vi "gen_logstring.vi"(11 "Movelist":T1[](array[typedef])) -> (3 "LogString":string)   [LabVIEW 2015]
uses:
  chess_moveinfo_cluster.ctl
  chess_piecetype_enum.ctl
  chess_teamcolor_enum.ctl
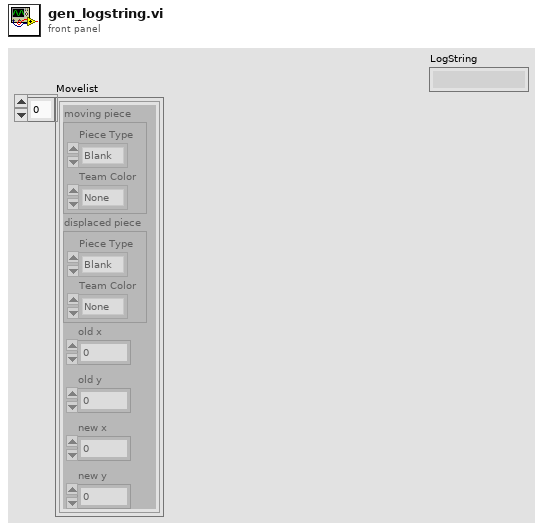
[diagram p1: front panel]
types:
  T1 = typedef "chess_moveinfo_cluster.ctl" = cluster{"moving piece":cluster{"Piece Type":T2, "Team Color":T3}, "displaced piece":cluster{"Piece Type":T2, "Team Color":T3}, "old x":i32, "old y":i32, "new x":i32, "new y":i32}
  T2 = typedef "chess_piecetype_enum.ctl" = enum16{"Blank", "Pawn", "Rook", "Knight", "Bishop", "Queen", "King"}
  T3 = typedef "chess_teamcolor_enum.ctl" = enum16{"None", "Red", "Blue"}
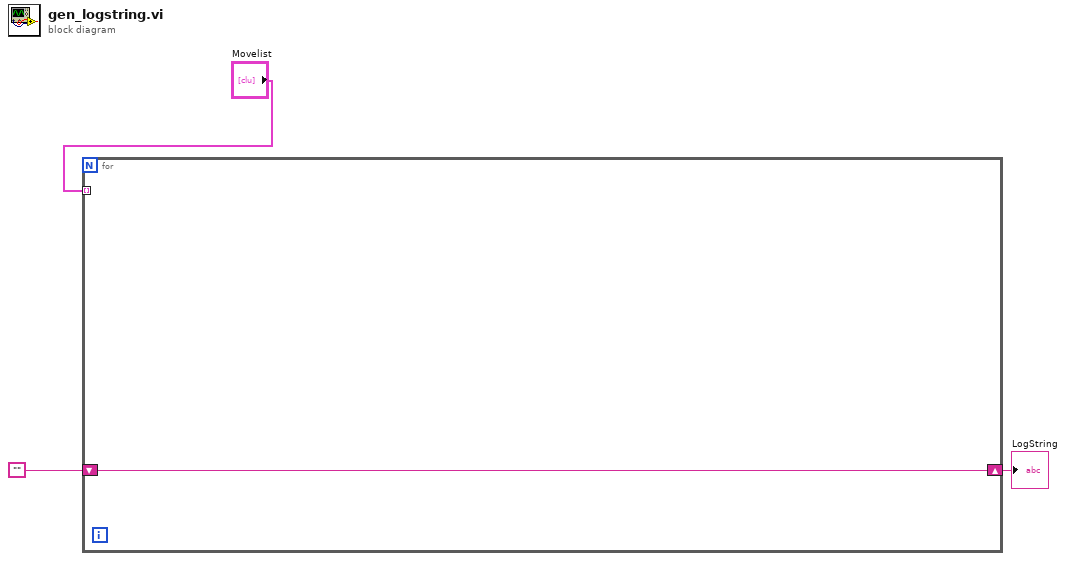
[diagram p0: block diagram]
diagram:
  n1 = for {
    tunnel: "Movelist" -> [_] mode=indexing
    shift-right: [w4] -> w1
    shift-left: "" -> [w4]
  }
  "LogString" <- w1
